vi "Parse Text-Tag-Text.vi"(8 "Error In":errorcluster) -> (0 "Error Out":errorcluster)   [LabVIEW 2017, in "Tests.lvlib" / "Parser.lvlib"]
uses:
  Parser.lvlib
  src/Mustache/Public/Tokens/Public/Text/Text.lvclass
  src/Mustache/Public/Tokens/Public/EscapedVariable/EscapedVariable.lvclass
  src/Mustache/Public/Tokens/Public/EscapedVariable/EscapedVariable.lvclass/EscapedVariable.ctl
  src/Mustache/Public/Readers/Public/String/String.lvclass
  D:/Users/cfield/Code/Field R&D Services/Mustache/feature-lv-original-parser/src/Mustache/Public/Readers/Public/Abstract/Abstract.lvclass
  <vilib>/addons/_JKI Toolkits/Caraya/classes/Test/Test.lvclass
  src/Mustache/Public/Parser/Parser.lvclass
  <vilib>/addons/_JKI Toolkits/Caraya/classes/Assert/Assert.lvclass
  src/Mustache/Public/Tokens/Public/Abstract/Abstract.lvclass
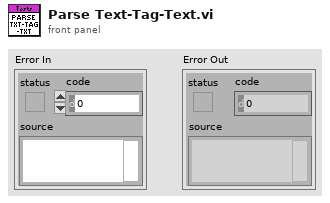
[diagram p1: front panel]
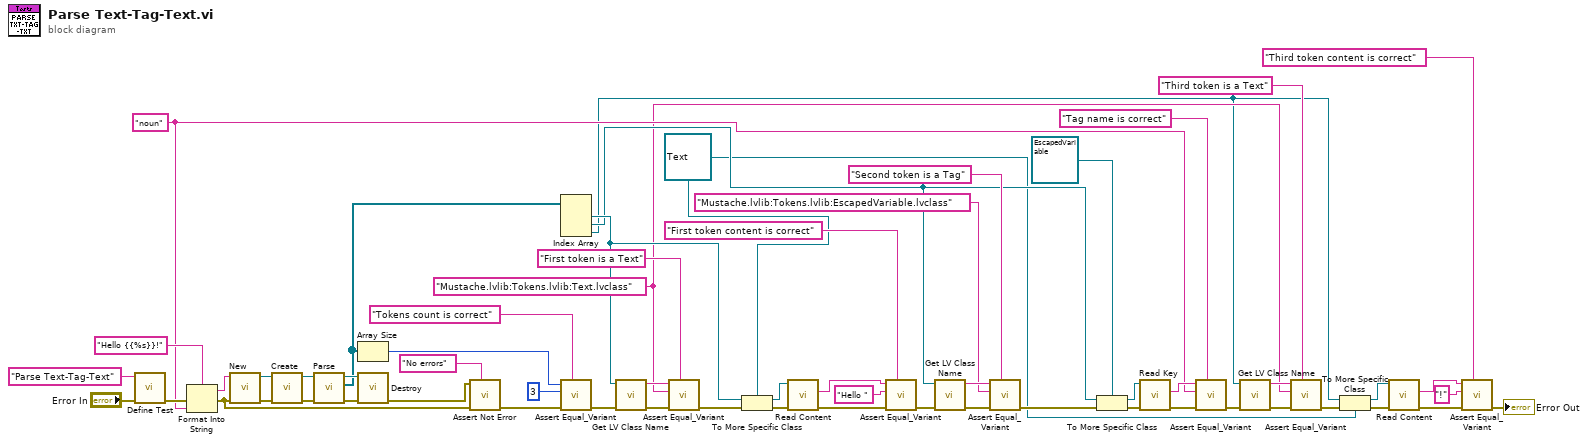
[diagram p0: block diagram]
diagram:
  w8 = refnum<class "Text.lvclass"> refnum ("Mustache.lvlib:Tokens.lvlib:Text.lvclass")
  w12 = "Mustache.lvlib:Tokens.lvlib:Text.lvclass"
  w17 = "noun" ("String")
  n1 = call <vilib>:"Define Test.vi"("error in (no error)"="Error In", "Label (VI Title)"="Parse Text-Tag-Text") -> ("error out"=w51:errorcluster)  [unwired: 9 in]
  n2 = Format Into String(format string="Hello {{%s}}!", error in=w51, w17) -> (resulting string=w32:string, error out=w34:errorcluster)  [unwired: 1 in]
  n3 = call "New.vi"("Error In"=w34, "String"=w32) -> ("Error Out"=w57:errorcluster, "String"=w58:refnum<class "String.lvclass">)  [unwired: 8 in]
  n4 = call "Create.vi"("Error In"=w57, "Reader"=w58) -> ("Error Out"=w56:errorcluster, "Parser"=w55:refnum<class "Parser.lvclass">)  [unwired: 8 in]
  n5 = call "Parse.vi"("Error In"=w56, "Parser In"=w55) -> ("Error Out"=w53:errorcluster, "Tokens"=w44:refnum<class "Abstract.lvclass">[], "Parser Out"=w54:refnum<class "Parser.lvclass">)  [unwired: 7 in]
  n6 = Array Size(array=w44) -> (size(s)=w47:i32)
  n7 = call "Destroy.vi"("Error In"=w53, "Parser"=w54) -> ("Error Out"=w52:errorcluster)  [unwired: 9 in]
  n8 = call <vilib>:"Assert Not Error.vi"("Label"="No errors", "error in (no error)"=w34, "Not Error?"=w52) -> ("error out"=w49:errorcluster)  [unwired: 8 in]
  n9 = Index Array(array=w44) -> (element #1=w30:refnum<class "Abstract.lvclass">, element #2=w22:refnum<class "Abstract.lvclass">, element #3=w9:refnum<class "Abstract.lvclass">)  [unwired: 3 in]
  n10 = call <vilib>:"Assert Equal_Variant.vi"("Label"="Tokens count is correct", "error in (no error)"=w49, "Y"=3 ("size(s)"), "X"=w47) -> ("error out"=w45:errorcluster)  [unwired: 7 in]
  n11 = call <vilib>:"Get LV Class Name.vi"("error in (no error)"=w45, "object"=w30) -> ("error out"=w43:errorcluster, "class name"=w42:string)  [unwired: 8 in]
  n12 = call <vilib>:"Assert Equal_Variant.vi"("Label"="First token is a Text", "error in (no error)"=w43, "Y"=w12, "X"=w42) -> ("error out"=w40:errorcluster)  [unwired: 7 in]
  n13 = To More Specific Class(target class=w8, reference=w30, error in=w40) -> (specific class reference=w28:refnum<class "Text.lvclass">, error out=w31:errorcluster)
  n14 = call "Read Content.vi"("Error In"=w31, "Text In"=w28) -> ("Error Out"=w29:errorcluster, "Content"=w26:string)  [unwired: 7 in, 1 out]
  n15 = call <vilib>:"Assert Equal_Variant.vi"("Label"="First token content is correct", "error in (no error)"=w29, "Y"="Hello ", "X"=w26) -> ("error out"=w27:errorcluster)  [unwired: 7 in]
  n16 = call <vilib>:"Get LV Class Name.vi"("error in (no error)"=w27, "object"=w22) -> ("error out"=w39:errorcluster, "class name"=w38:string)  [unwired: 8 in]
  n17 = call <vilib>:"Assert Equal_Variant.vi"("Label"="Second token is a Tag", "error in (no error)"=w39, "Y"="Mustache.lvlib:Tokens.lvlib:EscapedVariable.lvclass", "X"=w38) -> ("error out"=w36:errorcluster)  [unwired: 7 in]
  n18 = To More Specific Class(target class=refnum<class "EscapedVariable.lvclass"> refnum ("Mustache.lvlib:Tokens.lvlib:Tag.lvclass"), reference=w22, error in=w36) -> (specific class reference=w19:refnum<class "EscapedVariable.lvclass">, error out=w23:errorcluster)
  n19 = call "Read Key.vi"("Error In"=w23, "Tag In"=w19) -> ("Error Out"=w20:errorcluster, "Key"=w18:string)  [unwired: 7 in, 1 out]
  n20 = call <vilib>:"Assert Equal_Variant.vi"("Label"="Tag name is correct", "error in (no error)"=w20, "Y"=w17, "X"=w18) -> ("error out"=w15:errorcluster)  [unwired: 7 in]
  n21 = call <vilib>:"Get LV Class Name.vi"("error in (no error)"=w15, "object"=w9) -> ("error out"=w14:errorcluster, "class name"=w13:string)  [unwired: 8 in]
  n22 = call <vilib>:"Assert Equal_Variant.vi"("Label"="Third token is a Text", "error in (no error)"=w14, "Y"=w12, "X"=w13) -> ("error out"=w10:errorcluster)  [unwired: 7 in]
  n23 = To More Specific Class(target class=w8, reference=w9, error in=w10) -> (specific class reference=w6:refnum<class "Text.lvclass">, error out=w7:errorcluster)
  n24 = call "Read Content.vi"("Error In"=w7, "Text In"=w6) -> ("Error Out"=w5:errorcluster, "Content"=w2:string)  [unwired: 7 in, 1 out]
  n25 = call <vilib>:"Assert Equal_Variant.vi"("Label"="Third token content is correct", "error in (no error)"=w5, "Y"="!", "X"=w2) -> ("error out"=→"Error Out":errorcluster)  [unwired: 7 in]
